vi "CTRE_Phoenix_MotorControl_ConfigBaseSettings.vi"(6 "timeoutMs":i32=50, 7 "Force Write":bool, 8 "error in (no error)":errorcluster, 10 "Base Configurables":T1={"openLoopRamp"=0.0, "closedLoopRamp"=0.0, "peakOutputForward"=1.0, "peakOutputReverse"=-1.0, "nominalOutputForward"=0.0, "nominalOutputReverse"=0.0, "neutralDeadband"=0.04, "voltageCompSaturation"=0.0, "voltageMeasurementFilter"=32, "velocityMeasurementPeriod"=100, "velocityMeasurementWindow"=64, "forwardSoftLimitThreshold"=0, "reverseSoftLimitThreshold"=0, "forwardSoftLimitEnable"=FALSE, "reverseSoftLimitEnable"=FALSE, "slot0"={"P"=0.0, "I"=0.0, "D"=0.0, "F"=0.0, "integralZone"=0.0, "allowableClosedLoopError"=0, "maxIntegralAccumulator"=0.0, "closedLoopPeakOutput"=1.0, "closedLoopPeriod"=1}, "slot1"={"P"=0.0, "I"=0.0, "D"=0.0, "F"=0.0, "integralZone"=0.0, "allowableClosedLoopError"=0, "maxIntegralAccumulator"=0.0, "closedLoopPeakOutput"=1.0, "closedLoopPeriod"=1}, "slot2"={"P"=0.0, "I"=0.0, "D"=0.0, "F"=0.0, "integralZone"=0.0, "allowableClosedLoopError"=0, "maxIntegralAccumulator"=0.0, "closedLoopPeakOutput"=1.0, "closedLoopPeriod"=1}, "slot3"={"P"=0.0, "I"=0.0, "D"=0.0, "F"=0.0, "integralZone"=0.0, "allowableClosedLoopError"=0, "maxIntegralAccumulator"=0.0, "closedLoopPeakOutput"=1.0, "closedLoopPeriod"=1}, "auxPIDPolarity"=FALSE, "remoteFilter0"={"remoteSensorDeviceID"=0, "remoteSensorSource"=enum."Off"}, "remoteFilter1"={"remoteSensorDeviceID"=0, "remoteSensorSource"=enum."Off"}, "motionCruiseVelocity"=0, "motionAcceleration"=0, "motionProfileTrajectoryPeriod"=0, "feedbackNotContinuous"=FALSE, "remoteSensorClosedLoopDisableNeutralOnLOS"=FALSE, "clearPositionOnLimitF"=FALSE, "clearPositionOnLimitR"=FALSE, "clearPositionOnQuadIdx"=FALSE, "limitSwitchDisableNeutralOnLOS"=FALSE, "softLimitDisableNeutralOnLOS"=FALSE, "pulseWidthPeriod_EdgesPerRot"=1, "pulseWidthPeriod_FilterWindowSz"=1, "customParam"={"customParam0"=0, "customParam1"=0}, "trajectoryInterpolationEnable"=TRUE} {"velocityMeasurementPeriod" items=["Period_1ms"=1, "Period_2ms"=2, "Period_5ms"=5, "Period_10ms"=10, "Period_20ms"=20, "Period_25ms"=25, "Period_50ms"=50, "Period_100ms"=100]}, 11 "PhoenixMotorControlDevRef in":T7) -> (0 "error out":errorcluster, 3 "PhoenixMotorControlDevRef out":T7)   [LabVIEW 2020]
doc: "Sets the base motor controller configurations for the selected motor controller"
uses:
  <vilib>/Rock Robotics/WPI/MotorControl/WPI_MotorControlDeviceRef.ctl
  <vilib>/Rock Robotics/WPI/MotorControl/WPI_MotorControlType.ctl
  <vilib>/Rock Robotics/SystemInterfaces/DIO/FPGA_DIOPWMChannel.ctl
  <vilib>/Rock Robotics/WPI/PWM/WPI_PWMDeadband.ctl
  <vilib>/Rock Robotics/SystemInterfaces/DIO/FPGA_DIOChannel.ctl
  <vilib>/Rock Robotics/WPI/ThirdParty/Phoenix-LabVIEW/Motor Controller/Controls/CTRE_Phoenix_MotorControl_BaseConfigurables.ctl
  <vilib>/Rock Robotics/WPI/ThirdParty/Phoenix-LabVIEW/Motor Controller/Controls/CTRE_Phoenix_MotorControl_VelocityMeasurementPeriod.ctl
  <vilib>/Rock Robotics/WPI/ThirdParty/Phoenix-LabVIEW/Motor Controller/Controls/CTRE_Phoenix_MotorControl_SlotStructure.ctl
  <vilib>/Rock Robotics/WPI/ThirdParty/Phoenix-LabVIEW/Motor Controller/Controls/CTRE_Phoenix_MotorControl_FilterStruct.ctl
  <vilib>/Rock Robotics/WPI/ThirdParty/Phoenix-LabVIEW/Motor Controller/Controls/CTRE_Phoenix_MotorControl_RemoteSourceType.ctl
  <vilib>/Rock Robotics/WPI/ThirdParty/Phoenix-LabVIEW/Controls/CTRE_Phoenix_CustomParamConfiguration.ctl
panel:
  # "False: Primary Output = PID[0] + PID[1]  ---  Auxiliary Output = PID[0] - PID[1]\nTrue:  Primary Output = PID[0] - PID[1] --- Auxiliary Output = PID[0] + PID[1]"
  # "Enable the motion profile executor to perform linear interpolation between profile points.  Defaults to True."
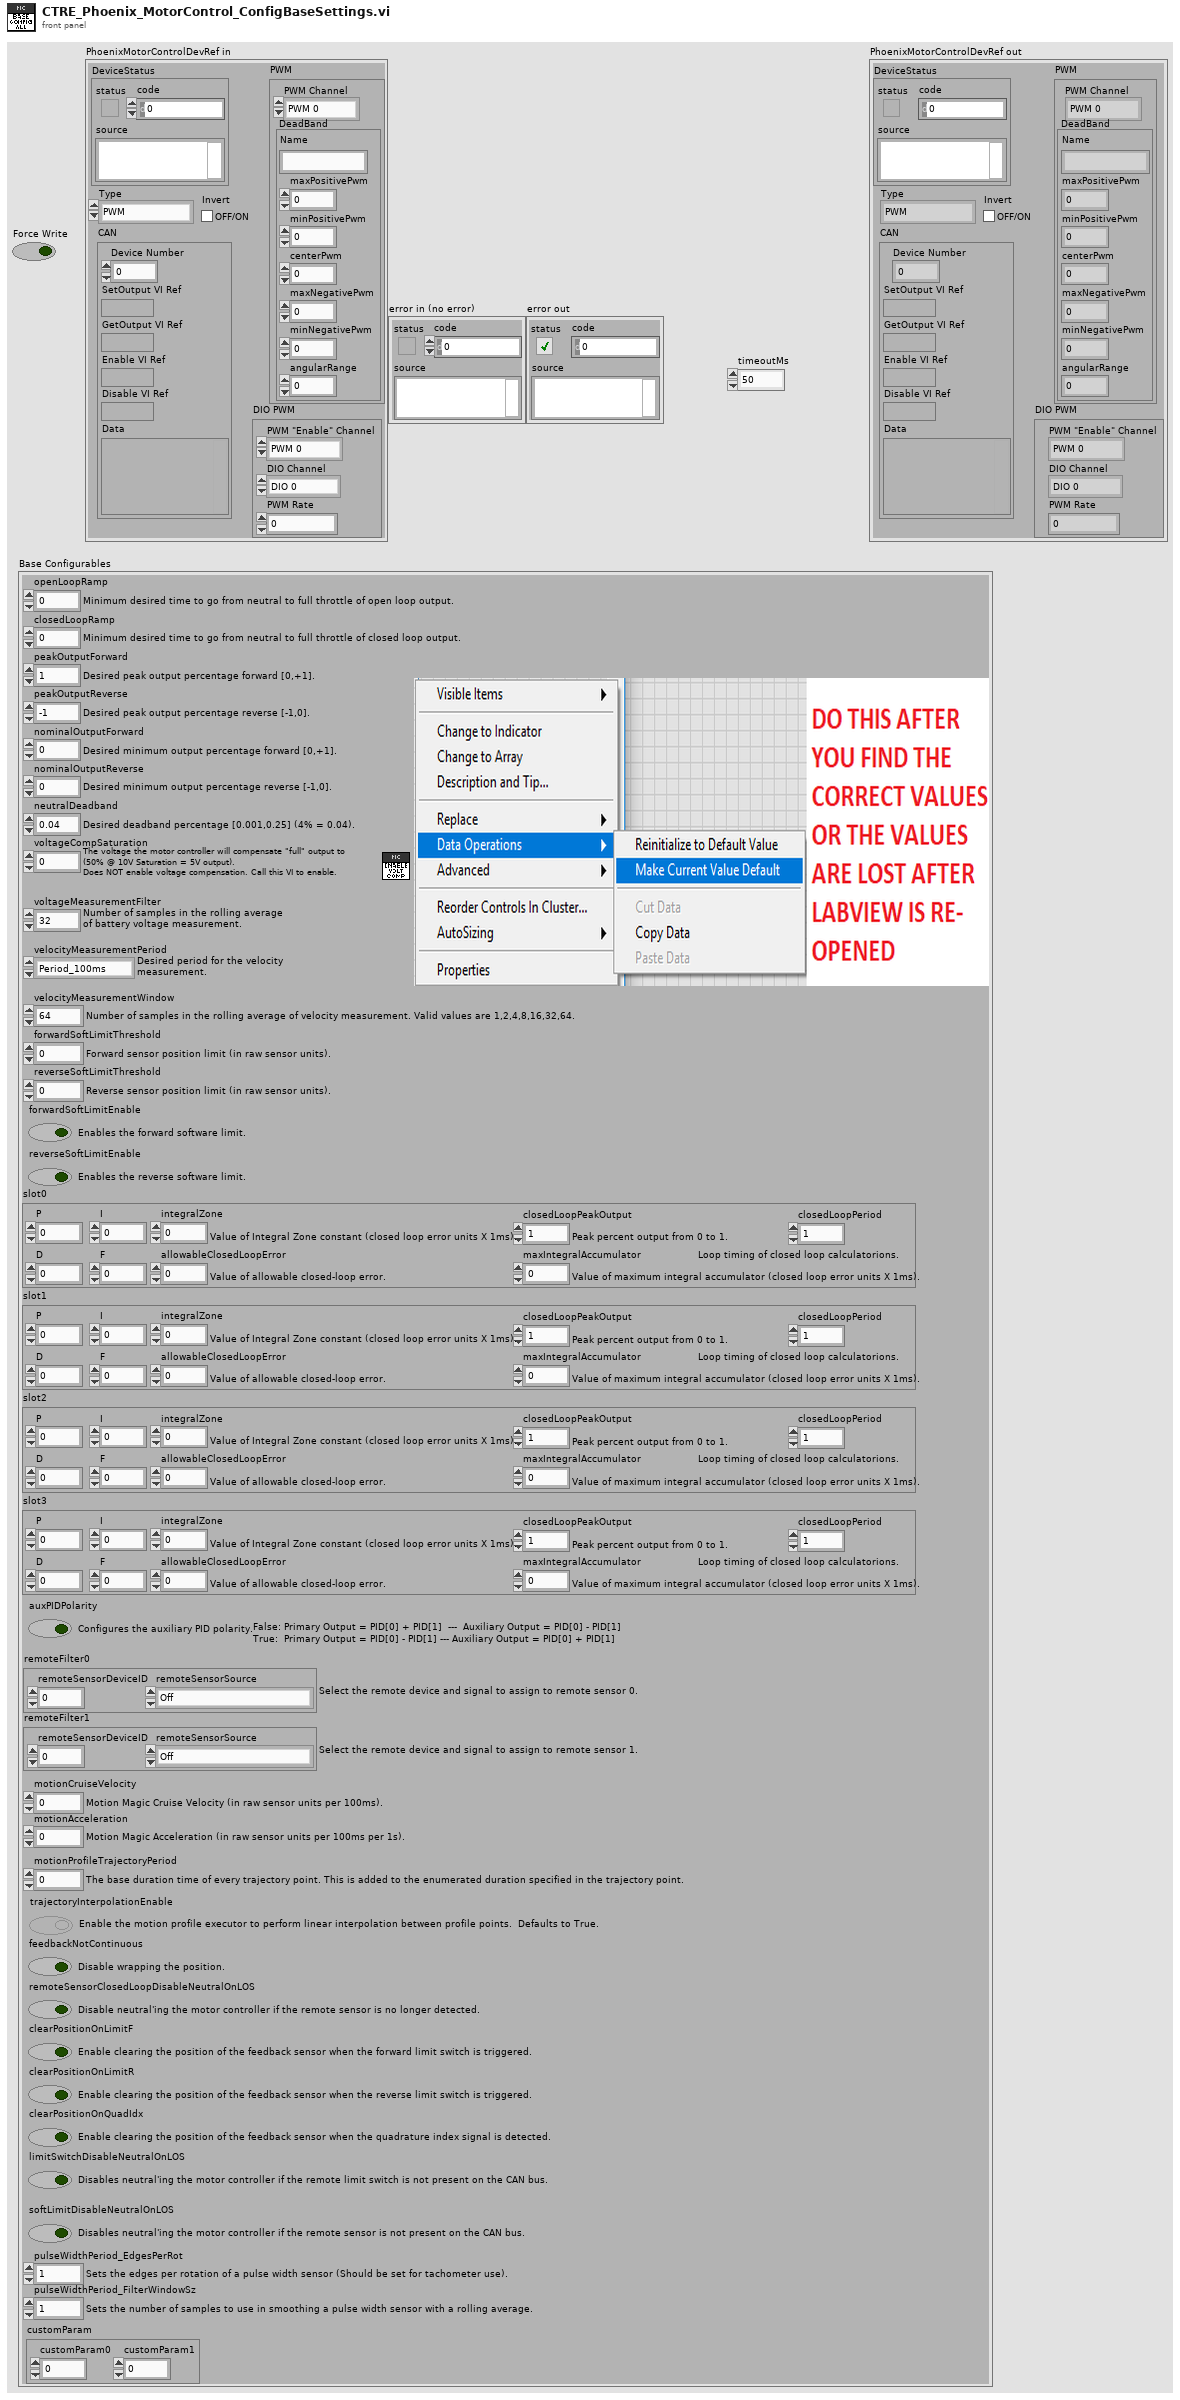
[diagram p1: front panel]
types:
  T1 = typedef "CTRE_Phoenix_MotorControl_BaseConfigurables.ctl" = cluster{"openLoopRamp":dbl, "closedLoopRamp":dbl, "peakOutputForward":dbl, "peakOutputReverse":dbl, "nominalOutputForward":dbl, "nominalOutputReverse":dbl, "neutralDeadband":dbl, "voltageCompSaturation":dbl, "voltageMeasurementFilter":i32, "velocityMeasurementPeriod":T2, "velocityMeasurementWindow":i32, "forwardSoftLimitThreshold":i32, "reverseSoftLimitThreshold":i32, "forwardSoftLimitEnable":bool, "reverseSoftLimitEnable":bool, "slot0":T3, "slot1":T3, "slot2":T3, "slot3":T3, "auxPIDPolarity":bool, "remoteFilter0":T4, "remoteFilter1":T4, "motionCruiseVelocity":i32, "motionAcceleration":i32, "motionProfileTrajectoryPeriod":i32, "feedbackNotContinuous":bool, "remoteSensorClosedLoopDisableNeutralOnLOS":bool, "clearPositionOnLimitF":bool, "clearPositionOnLimitR":bool, "clearPositionOnQuadIdx":bool, "limitSwitchDisableNeutralOnLOS":bool, "softLimitDisableNeutralOnLOS":bool, "pulseWidthPeriod_EdgesPerRot":i32, "pulseWidthPeriod_FilterWindowSz":i32, "customParam":T6, "trajectoryInterpolationEnable":bool}
  T2 = typedef "CTRE_Phoenix_MotorControl_VelocityMeasurementPeriod.ctl" = u16
  T3 = typedef "CTRE_Phoenix_MotorControl_SlotStructure.ctl" = cluster{"P":dbl, "I":dbl, "D":dbl, "F":dbl, "integralZone":dbl, "allowableClosedLoopError":i32, "maxIntegralAccumulator":dbl, "closedLoopPeakOutput":dbl, "closedLoopPeriod":i32}
  T4 = typedef "CTRE_Phoenix_MotorControl_FilterStruct.ctl" = cluster{"remoteSensorDeviceID":u8, "remoteSensorSource":T5}
  T5 = typedef "CTRE_Phoenix_MotorControl_RemoteSourceType.ctl" = enum16{"Off", "Talon SRX Selected Sensor", "Pigeon IMU Yaw", "Pigeon IMU Pitch", "Pigeon IMU Roll", "CANifier Quadrature", "CANifier PWM Input 0", "CANifier PWM Input 1", "CANifier PWM Input 2", "CANifier PWM Input 3", "Gadgeteer Pigeon Yaw", "Gadgeteer Pigeon Pitch", "Gadgeteer Pigeon Roll", "CANCoder"}
  T6 = typedef "CTRE_Phoenix_CustomParamConfiguration.ctl" = cluster{"customParam0":i32, "customParam1":i32}
  T7 = typedef "WPI_MotorControlDeviceRef.ctl" = cluster{"DeviceStatus":errorcluster, "Type":T8, "PWM":cluster{"PWM Channel":T9, "DeadBand":T10}, "CAN":cluster{"Device Number":u8, "SetOutput VI Ref":variant, "GetOutput VI Ref":variant, "Enable VI Ref":variant, "Disable VI Ref":variant, "Data":variant}, "Invert":bool, "DIO PWM":cluster{"PWM \"Enable\" Channel":T9, "DIOChannel":T11, "PWM Rate":dbl}}
  T8 = typedef "WPI_MotorControlType.ctl" = enum16{"PWM", "CAN", "DIO PWM"}
  T9 = typedef "FPGA_DIOPWMChannel.ctl" = enum8{"PWM 0", "PWM 1", "PWM 2", "PWM 3", "PWM 4", "PWM 5", "PWM 6", "PWM 7", "PWM 8", "PWM 9", "PWM MXP 0", "PWM MXP 1", "PWM MXP 2", "PWM MXP 3", "PWM MXP 4", "PWM MXP 5", "PWM MXP 6", "PWM MXP 7", "PWM MXP 8", "PWM MXP 9", "Invalid"}
  T10 = typedef "WPI_PWMDeadband.ctl" = cluster{"Name":string, "maxPositivePwm":i32, "minPositivePwm":i32, "centerPwm":i32, "maxNegativePwm":i32, "minNegativePwm":i32, "angularRange":u16}
  T11 = typedef "FPGA_DIOChannel.ctl" = enum8{"DIO 0", "DIO 1", "DIO 2", "DIO 3", "DIO 4", "DIO 5", "DIO 6", "DIO 7", "DIO 8", "DIO 9", "DIO MXP 0", "DIO MXP 1", "DIO MXP 2", "DIO MXP 3", "DIO MXP 4", "DIO MXP 5", "DIO MXP 6", "DIO MXP 7", "DIO MXP 8", "DIO MXP 9", "DIO MXP 10", "DIO MXP 11", "DIO MXP 12", "DIO MXP 13", "DIO MXP 14", "DIO MXP 15", "SPI Port CS1", "SPI Port CS2", "SPI Port CS3", "SPI Port MISO", "SPI Port MOSI", "Invalid"}
  T12 = cluster{"openLoopRamp":bool, "closedLoopRamp":bool, "peakOutputForward":bool, "peakOutputReverse":bool, "nominalOutputForward":bool, "nominalOutputReverse":bool, "neutralDeadband":bool, "voltageCompSaturation":bool, "voltageMeasurementFilter":bool, "velocityMeasurementPeriod":bool, "velocityMeasurementWindow":bool, "forwardSoftLimitThreshold":bool, "reverseSoftLimitThreshold":bool, "forwardSoftLimitEnable":bool, "reverseSoftLimitEnable":bool, "slot0":cluster{"P":bool, "I":bool, "D":bool, "F":bool, "integralZone":bool, "allowableClosedLoopError":bool, "maxIntegralAccumulator":bool, "closedLoopPeakOutput":bool, "closedLoopPeriod":bool}, "slot1":cluster{"P":bool, "I":bool, "D":bool, "F":bool, "integralZone":bool, "allowableClosedLoopError":bool, "maxIntegralAccumulator":bool, "closedLoopPeakOutput":bool, "closedLoopPeriod":bool}, "slot2":cluster{"P":bool, "I":bool, "D":bool, "F":bool, "integralZone":bool, "allowableClosedLoopError":bool, "maxIntegralAccumulator":bool, "closedLoopPeakOutput":bool, "closedLoopPeriod":bool}, "slot3":cluster{"P":bool, "I":bool, "D":bool, "F":bool, "integralZone":bool, "allowableClosedLoopError":bool, "maxIntegralAccumulator":bool, "closedLoopPeakOutput":bool, "closedLoopPeriod":bool}, "auxPIDPolarity":bool, "remoteFilter0":cluster{"remoteSensorDeviceID":bool, "remoteSensorSource":bool}, "remoteFilter1":cluster{"remoteSensorDeviceID":bool, "remoteSensorSource":bool}, "motionCruiseVelocity":bool, "motionAcceleration":bool, "motionProfileTrajectoryPeriod":bool, "feedbackNotContinuous":bool, "remoteSensorClosedLoopDisableNeutralOnLOS":bool, "clearPositionOnLimitF":bool, "clearPositionOnLimitR":bool, "clearPositionOnQuadIdx":bool, "limitSwitchDisableNeutralOnLOS":bool, "softLimitDisableNeutralOnLOS":bool, "pulseWidthPeriod_EdgesPerRot":bool, "pulseWidthPeriod_FilterWindowSz":bool, "customParam":cluster{"customParam0":bool, "customParam1":bool}, "trajectoryInterpolationEnable":bool}
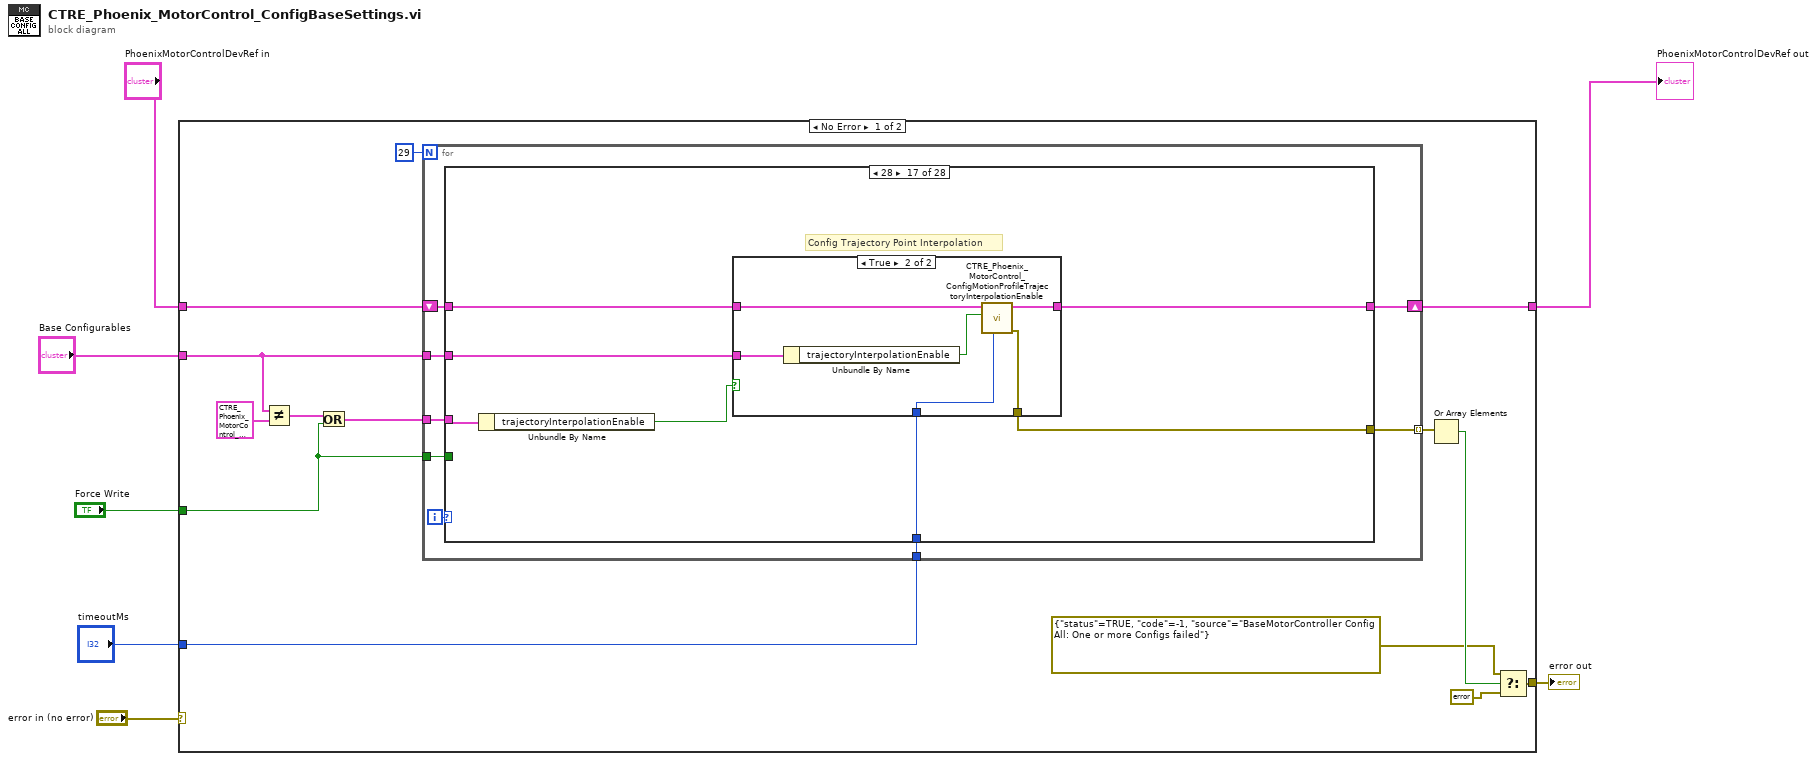
[diagram p0: block diagram]
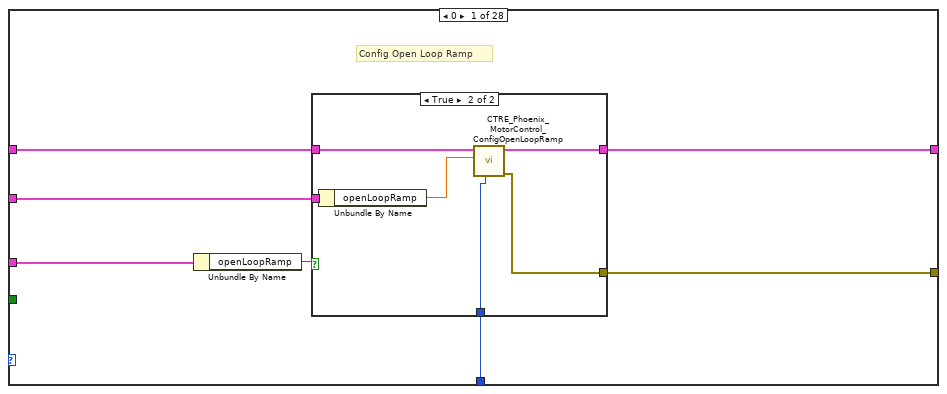
[diagram p2: hidden frame]
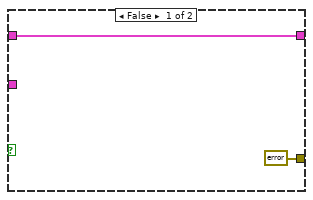
[diagram p3: hidden frame]
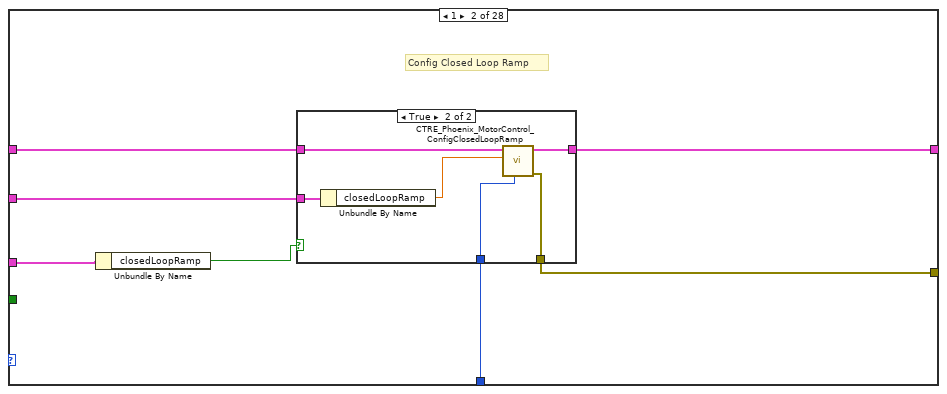
[diagram p4: hidden frame]
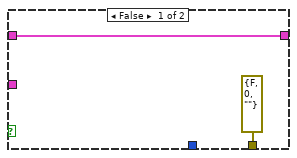
[diagram p5: hidden frame]
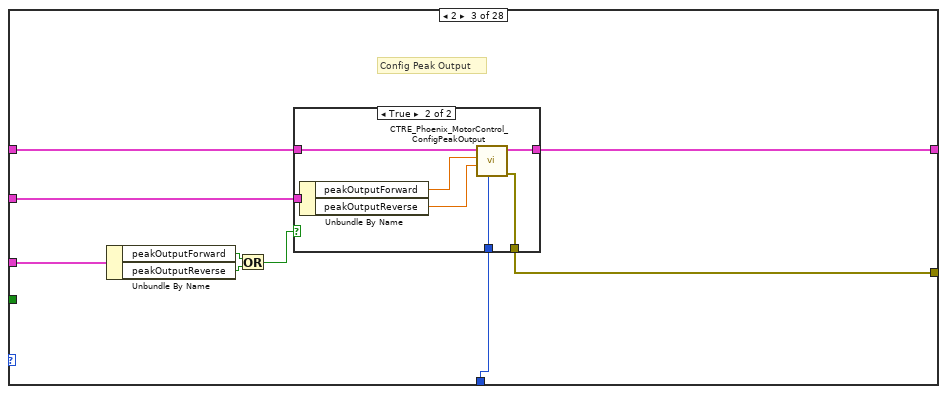
[diagram p6: hidden frame]
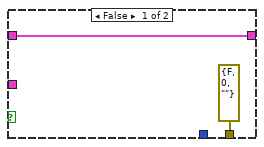
[diagram p7: hidden frame]
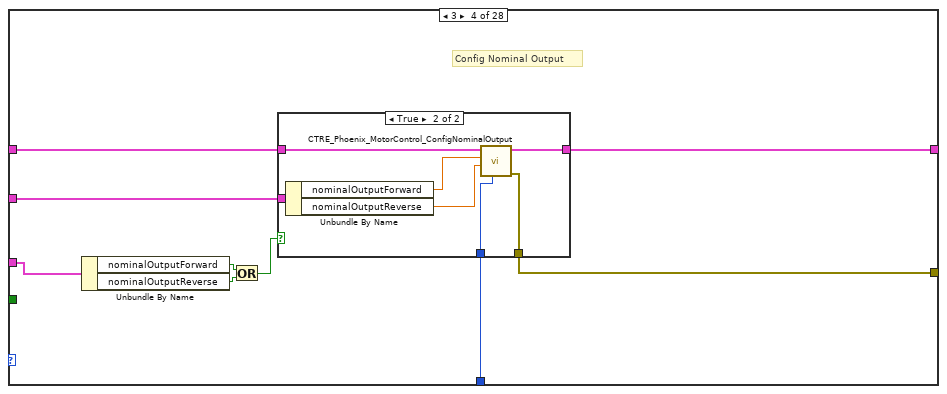
[diagram p8: hidden frame]
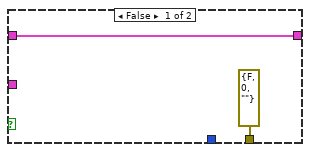
[diagram p9: hidden frame]
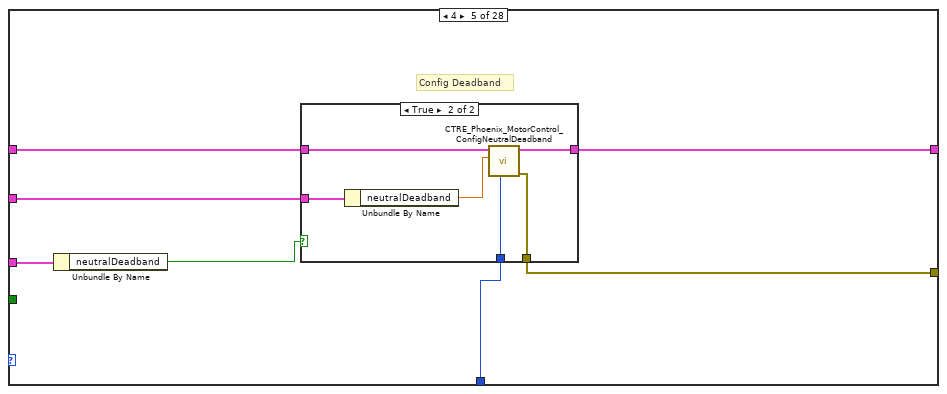
[diagram p10: hidden frame]
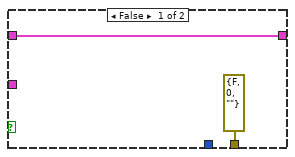
[diagram p11: hidden frame]
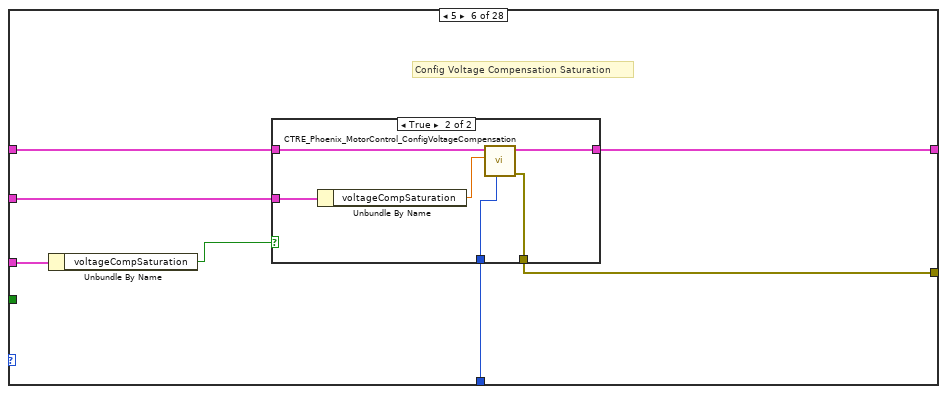
[diagram p12: hidden frame]
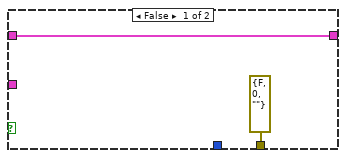
[diagram p13: hidden frame]
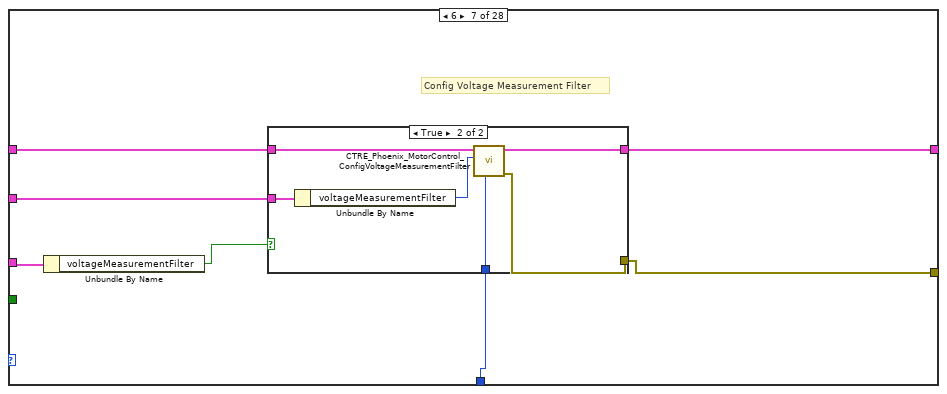
[diagram p14: hidden frame]
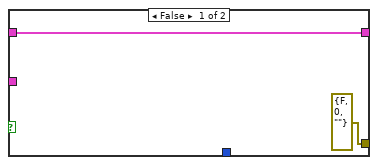
[diagram p15: hidden frame]
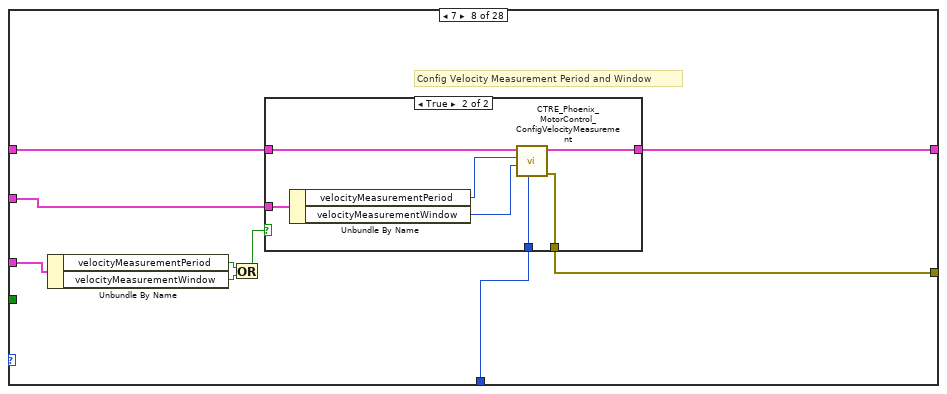
[diagram p16: hidden frame]
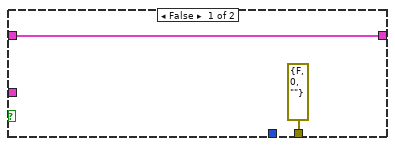
[diagram p17: hidden frame]
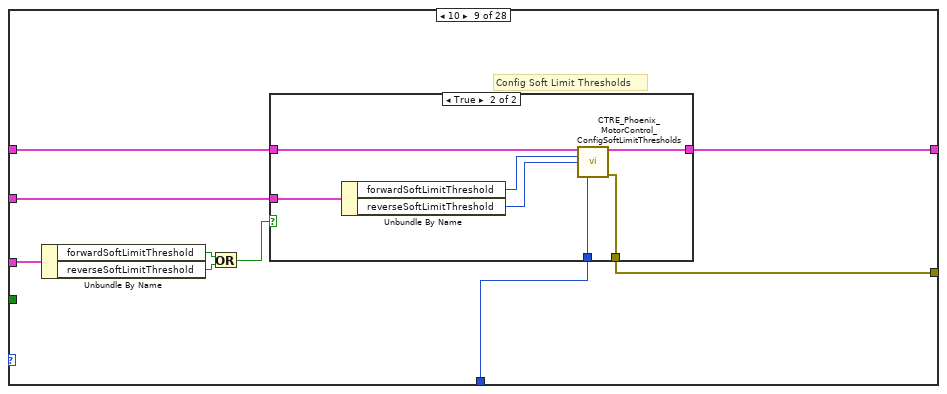
[diagram p18: hidden frame]
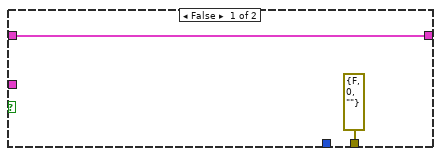
[diagram p19: hidden frame]
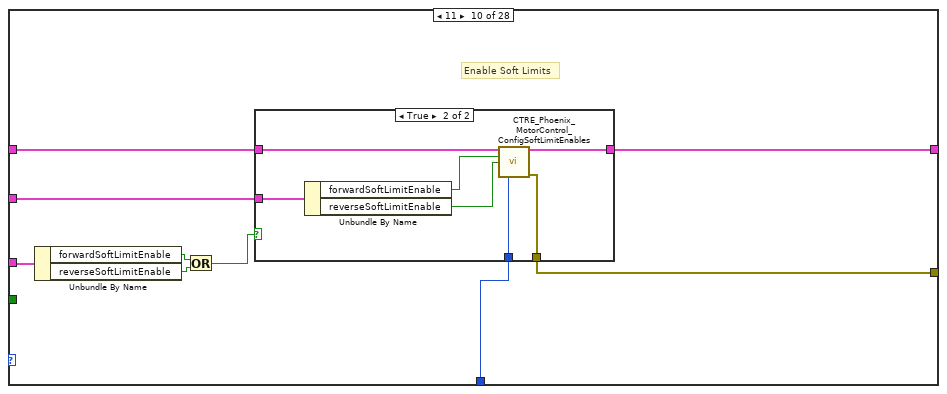
[diagram p20: hidden frame]
diagram:
  n1 = case shown="No Error" "error in (no error)" {
    selector: "error in (no error)" -> [_ w467]
    tunnel: "timeoutMs" -> [w19 _]
    tunnel: [w18 w468] -> w6
    tunnel: "PhoenixMotorControlDevRef in" -> [w17 w468]
    tunnel: "Base Configurables" -> [w16 _]
    tunnel: "Force Write" -> [w12 _]
    tunnel: [w8 w467] -> w1
    frame No Error {
      n2 = Not Equal?(x=w16, y=T1 {"openLoopRamp"=0.0, "closedLoopRamp"=0.0, "peakOutputForward"=1.0, "peakOutputReverse"=-1.0, "nominalOutputForward"=0.0, "nominalOutputReverse"=0.0, "neutralDeadband"=0.04, "voltageCompSaturation"=0.0, "voltageMeasurementFilter"=32, "velocityMeasurementPeriod"=100, "velocityMeasurementWindow"=64, "forwardSoftLimitThreshold"=0, "reverseSoftLimitThreshold"=0, "forwardSoftLimitEnable"=FALSE, "reverseSoftLimitEnable"=FALSE, "slot0"={"P"=0.0, "I"=0.0, "D"=0.0, "F"=0.0, "integralZone"=0.0, "allowableClosedLoopError"=0, "maxIntegralAccumulator"=0.0, "closedLoopPeakOutput"=1.0, "closedLoopPeriod"=1}, "slot1"={"P"=0.0, "I"=0.0, "D"=0.0, "F"=0.0, "integralZone"=0.0, "allowableClosedLoopError"=0, "maxIntegralAccumulator"=0.0, "closedLoopPeakOutput"=1.0, "closedLoopPeriod"=1}, "slot2"={"P"=0.0, "I"=0.0, "D"=0.0, "F"=0.0, "integralZone"=0.0, "allowableClosedLoopError"=0, "maxIntegralAccumulator"=0.0, "closedLoopPeakOutput"=1.0, "closedLoopPeriod"=1}, "slot3"={"P"=0.0, "I"=0.0, "D"=0.0, "F"=0.0, "integralZone"=0.0, "allowableClosedLoopError"=0, "maxIntegralAccumulator"=0.0, "closedLoopPeakOutput"=1.0, "closedLoopPeriod"=1}, "auxPIDPolarity"=FALSE, "remoteFilter0"={"remoteSensorDeviceID"=0, "remoteSensorSource"=enum."Off"}, "remoteFilter1"={"remoteSensorDeviceID"=0, "remoteSensorSource"=enum."Off"}, "motionCruiseVelocity"=0, "motionAcceleration"=0, "motionProfileTrajectoryPeriod"=0, "feedbackNotContinuous"=FALSE, "remoteSensorClosedLoopDisableNeutralOnLOS"=FALSE, "clearPositionOnLimitF"=FALSE, "clearPositionOnLimitR"=FALSE, "clearPositionOnQuadIdx"=FALSE, "limitSwitchDisableNeutralOnLOS"=FALSE, "softLimitDisableNeutralOnLOS"=FALSE, "pulseWidthPeriod_EdgesPerRot"=1, "pulseWidthPeriod_FilterWindowSz"=1, "customParam"={"customParam0"=0, "customParam1"=0}, "trajectoryInterpolationEnable"=TRUE}) -> (x != y?=w14:T12)
      n3 = Or(x=w14, y=w12) -> (x .or. y?=w13:T12)
      n4 = for {
        N: 29 -> [_]
        tunnel: w19 -> [w27]
        tunnel: w16 -> [w26]
        shift-right: [w28] -> w18
        shift-left: w17 -> [w29]
        tunnel: [w24] -> w20 mode=indexing
        tunnel: w13 -> [w23]
        tunnel: w12 -> [w22]
        i -> [w25]
        n5 = case shown="28" w25 {
          tunnel: w29 -> [w35 w49 w67 w85 w101 w116 w131 w148 w166 w185 w202 w226 w243 w262 w281 w297 w312 w327 w342 w357 w372 w387 w402 w417 w432 w447 w463 w466]
          tunnel: [w34 w50 w66 w84 w100 w115 w130 w147 w165 w184 w201 w225 w242 w263 w280 w296 w311 w326 w341 w356 w371 w386 w400 w416 w431 w446 w462 w466] -> w28
          tunnel: w27 -> [w33 w48 w64 w82 w99 w114 w129 w146 w164 w182 w199 w224 w241 w260 w279 w295 w310 w325 w340 w355 w370 w385 w401 w415 w429 w445 w461 _]
          tunnel: w26 -> [w36 w51 w68 w86 w102 w117 w132 w149 w167 w183 w204 w227 w244 w261 w282 w298 w313 w328 w343 w358 w373 w388 w403 w418 w433 w448 w464 _]
          tunnel: [w32 w47 w65 w83 w98 w113 w128 w145 w163 w181 w197 w223 w240 w259 w278 w294 w309 w324 w339 w354 w369 w384 w399 w414 w430 w444 w457 errorcluster {"status"=FALSE, "code"=0, "source"=""} ("error out")] -> w24
          tunnel: w23 -> [w31 w46 w63 w81 w97 w112 w127 w144 w162 w180 _ w222 w239 w258 w277 w293 w308 w323 w338 w353 w368 w383 w398 w413 w428 w442 _ _]
          tunnel: w22 -> [_ _ _ _ _ _ _ _ _ _ w195 _ _ _ _ _ _ _ _ _ _ _ _ _ _ _ _ _]
          frame 0 {
            # "Config Open Loop Ramp"
            n6 = Unbundle By Name(w31) -> ("openLoopRamp"=w30:bool)
            n7 = case shown="True" w30 {
              tunnel: w36 -> [_ w44]
              tunnel: w35 -> [w38 w43]
              tunnel: [w38 w42] -> w34
              tunnel: w33 -> [_ w40]
              tunnel: [errorcluster {"status"=FALSE, "code"=0, "source"=""} ("error out") w39] -> w32
              frame False {
              }
              frame True {
                n8 = Unbundle By Name(w44) -> ("openLoopRamp"=w41:dbl)
                n9 = call <vilib>:"CTRE_Phoenix_MotorControl_ConfigOpenLoopRamp.vi"("timeoutMs"=w40, "secondsFromNeutralToFull"=w41, "PhoenixMotorControlDevRef"=w43) -> ("error out"=w39:errorcluster, "PhoenixMotorControlDevRef"=w42:T7)  [unwired: 7 in]
              }
            }
          }
          frame 1 {
            # "Config Closed Loop Ramp"
            n10 = Unbundle By Name(w46) -> ("closedLoopRamp"=w45:bool)
            n11 = case shown="True" w45 {
              tunnel: w51 -> [_ w59]
              tunnel: [w53 w58] -> w50
              tunnel: w49 -> [w53 w57]
              tunnel: w48 -> [_ w55]
              tunnel: [errorcluster {"status"=FALSE, "code"=0, "source"=""} ("error out") w54] -> w47
              frame False {
              }
              frame True {
                n12 = Unbundle By Name(w59) -> ("closedLoopRamp"=w56:dbl)
                n13 = call <vilib>:"CTRE_Phoenix_MotorControl_ConfigClosedLoopRamp.vi"("timeoutMs"=w55, "secondsFromNeutralToFull"=w56, "PhoenixMotorControlDevRef"=w57) -> ("error out"=w54:errorcluster, "PhoenixMotorControlDevRef"=w58:T7)  [unwired: 7 in]
              }
            }
          }
          frame 2 {
            # "Config Peak Output"
            n14 = Unbundle By Name(w63) -> ("peakOutputForward"=w61:bool, "peakOutputReverse"=w62:bool)
            n15 = Or(x=w61, y=w62) -> (x .or. y?=w60:bool)
            n16 = case shown="True" w60 {
              tunnel: w68 -> [_ w77]
              tunnel: w67 -> [w70 w76]
              tunnel: [w70 w75] -> w66
              tunnel: [errorcluster {"status"=FALSE, "code"=0, "source"=""} ("error out") w72] -> w65
              tunnel: w64 -> [_ w71]
              frame False {
              }
              frame True {
                n17 = Unbundle By Name(w77) -> ("peakOutputForward"=w74:dbl, "peakOutputReverse"=w73:dbl)
                n18 = call <vilib>:"CTRE_Phoenix_MotorControl_ConfigPeakOutput.vi"("timeoutMs"=w71, "Reverse Peak Percent Output"=w73, "Forward Peak Percent Output"=w74, "PhoenixMotorControlDevRef"=w76) -> ("error out"=w72:errorcluster, "PhoenixMotorControlDevRef"=w75:T7)  [unwired: 6 in]
              }
            }
          }
          frame 3 {
            # "Config Nominal Output"
            n19 = Unbundle By Name(w81) -> ("nominalOutputForward"=w79:bool, "nominalOutputReverse"=w80:bool)
            n20 = Or(x=w79, y=w80) -> (x .or. y?=w78:bool)
            n21 = case shown="True" w78 {
              tunnel: w86 -> [_ w95]
              tunnel: w85 -> [w88 w94]
              tunnel: [w88 w93] -> w84
              tunnel: [errorcluster {"status"=FALSE, "code"=0, "source"=""} ("error out") w90] -> w83
              tunnel: w82 -> [_ w89]
              frame False {
              }
              frame True {
                n22 = Unbundle By Name(w95) -> ("nominalOutputForward"=w92:dbl, "nominalOutputReverse"=w91:dbl)
                n23 = call <vilib>:"CTRE_Phoenix_MotorControl_ConfigNominalOutput.vi"("timeoutMs"=w89, "Reverse Nominal Percent Output"=w91, "Forward Nominal Percent Output"=w92, "PhoenixMotorControlDevRef"=w94) -> ("error out"=w90:errorcluster, "PhoenixMotorControlDevRef"=w93:T7)  [unwired: 6 in]
              }
            }
          }
          frame 4 {
            # "Config Deadband"
            n24 = Unbundle By Name(w97) -> ("neutralDeadband"=w96:bool)
            n25 = case shown="True" w96 {
              tunnel: w102 -> [_ w110]
              tunnel: w101 -> [w104 w109]
              tunnel: [w104 w108] -> w100
              tunnel: w99 -> [_ w106]
              tunnel: [errorcluster {"status"=FALSE, "code"=0, "source"=""} ("error out") w105] -> w98
              frame False {
              }
              frame True {
                n26 = Unbundle By Name(w110) -> ("neutralDeadband"=w107:dbl)
                n27 = call <vilib>:"CTRE_Phoenix_MotorControl_ConfigNeutralDeadband.vi"("timeoutMs"=w106, "Percent Deadband"=w107, "PhoenixMotorControlDevRef"=w109) -> ("error out"=w105:errorcluster, "PhoenixMotorControlDevRef"=w108:T7)  [unwired: 7 in]
              }
            }
          }
          frame 5 {
            # "Config Voltage Compensation Saturation"
            n28 = Unbundle By Name(w112) -> ("voltageCompSaturation"=w111:bool)
            n29 = case shown="True" w111 {
              tunnel: w117 -> [_ w125]
              tunnel: w116 -> [w119 w124]
              tunnel: [w119 w123] -> w115
              tunnel: w114 -> [_ w121]
              tunnel: [errorcluster {"status"=FALSE, "code"=0, "source"=""} ("error out") w120] -> w113
              frame False {
              }
              frame True {
                n30 = Unbundle By Name(w125) -> ("voltageCompSaturation"=w122:dbl)
                n31 = call <vilib>:"CTRE_Phoenix_MotorControl_ConfigVoltageCompensation.vi"("timeoutMs"=w121, "Saturation Voltage"=w122, "PhoenixMotorControlDevRef"=w124) -> ("error out"=w120:errorcluster, "PhoenixMotorControlDevRef"=w123:T7)  [unwired: 7 in]
              }
            }
          }
          frame 6 {
            # "Config Voltage Measurement Filter"
            n32 = Unbundle By Name(w127) -> ("voltageMeasurementFilter"=w126:bool)
            n33 = case shown="True" w126 {
              tunnel: w132 -> [_ w140]
              tunnel: w131 -> [w134 w139]
              tunnel: [w134 w138] -> w130
              tunnel: w129 -> [_ w136]
              tunnel: [errorcluster {"status"=FALSE, "code"=0, "source"=""} ("error out") w135] -> w128
              frame False {
              }
              frame True {
                n34 = Unbundle By Name(w140) -> ("voltageMeasurementFilter"=w137:i32)
                n35 = call <vilib>:"CTRE_Phoenix_MotorControl_ConfigVoltageMeasurementFilter.vi"("timeoutMs"=w136, "filterWindowSamples"=w137, "PhoenixMotorControlDevRef"=w139) -> ("error out"=w135:errorcluster, "PhoenixMotorControlDevRef"=w138:T7)  [unwired: 7 in]
              }
            }
          }
          frame 7 {
            # "Config Velocity Measurement Period and Window"
            n36 = Unbundle By Name(w144) -> ("velocityMeasurementPeriod"=w142:bool, "velocityMeasurementWindow"=w143:bool)
            n37 = Or(x=w142, y=w143) -> (x .or. y?=w141:bool)
            n38 = case shown="True" w141 {
              tunnel: w149 -> [_ w158]
              tunnel: w148 -> [w151 w157]
              tunnel: [w151 w156] -> w147
              tunnel: w146 -> [_ w153]
              tunnel: [errorcluster {"status"=FALSE, "code"=0, "source"=""} ("error out") w152] -> w145
              frame False {
              }
              frame True {
                n39 = Unbundle By Name(w158) -> ("velocityMeasurementPeriod"=w155:T2, "velocityMeasurementWindow"=w154:i32)
                n40 = call <vilib>:"CTRE_Phoenix_MotorControl_ConfigVelocityMeasurement.vi"("timeoutMs"=w153, "Window Size"=w154, "Velocity Measurement Period"=w155, "PhoenixMotorControlDevRef"=w157) -> ("error out"=w152:errorcluster, "PhoenixMotorControlDevRef"=w156:T7)  [unwired: 6 in]
              }
            }
          }
          frame 10 {
            # "Config Soft Limit Thresholds"
            n41 = Unbundle By Name(w162) -> ("forwardSoftLimitThreshold"=w160:bool, "reverseSoftLimitThreshold"=w161:bool)
            n42 = Or(x=w160, y=w161) -> (x .or. y?=w159:bool)
            n43 = case shown="True" w159 {
              tunnel: w167 -> [_ w176]
              tunnel: w166 -> [w169 w175]
              tunnel: [w169 w174] -> w165
              tunnel: w164 -> [_ w171]
              tunnel: [errorcluster {"status"=FALSE, "code"=0, "source"=""} ("error out") w170] -> w163
              frame False {
              }
              frame True {
                n44 = Unbundle By Name(w176) -> ("forwardSoftLimitThreshold"=w173:i32, "reverseSoftLimitThreshold"=w172:i32)
                n45 = call <vilib>:"CTRE_Phoenix_MotorControl_ConfigSoftLimitThresholds.vi"("PhoenixMotorControlDevRef"=w175, "Forward Soft Limit"=w173, "Reverse Soft Limit"=w172, "timeoutMs"=w171) -> ("PhoenixMotorControlDevRef"=w174:T7, "error out"=w170:errorcluster)  [unwired: 10 in]
              }
            }
          }
          frame 11 {
            # "Enable Soft Limits"
            n46 = Unbundle By Name(w180) -> ("forwardSoftLimitEnable"=w178:bool, "reverseSoftLimitEnable"=w179:bool)
            n47 = Or(x=w178, y=w179) -> (x .or. y?=w177:bool)
            n48 = case shown="True" w177 {
              tunnel: w185 -> [w187 w194]
              tunnel: [w187 w193] -> w184
              tunnel: w183 -> [_ w192]
              tunnel: w182 -> [_ w189]
              tunnel: [errorcluster {"status"=FALSE, "code"=0, "source"=""} ("error out") w188] -> w181
              frame False {
              }
              frame True {
                n49 = Unbundle By Name(w192) -> ("forwardSoftLimitEnable"=w191:bool, "reverseSoftLimitEnable"=w190:bool)
                n50 = call <vilib>:"CTRE_Phoenix_MotorControl_ConfigSoftLimitEnables.vi"("PhoenixMotorControlDevRef"=w194, "Forward Soft Limit Enable"=w191, "Reverse Soft Limit Enable"=w190, "timeoutMs"=w189) -> ("PhoenixMotorControlDevRef"=w193:T7, "error out"=w188:errorcluster)  [unwired: 10 in]
              }
            }
          }
          frame 12 {
            # "Configure the 4 slots"
            n51 = for {
              N: 4 -> [_]
              tunnel: w204 -> [w212]
              shift-right: [w211] -> w201
              shift-left: w202 -> [w209]
              tunnel: [w206] -> w200 mode=indexing
              tunnel: w199 -> [w210]
              tunnel: w195 -> [w205]
              i -> [w207]
              n52 = case shown="3" w207 {
                tunnel: w212 -> [w214 w216 w218 w220]
                tunnel: [w213 w215 w217 w219] -> w208
                frame 3 {
                  n53 = Unbundle By Name(w214) -> ("slot3"=w213:T3)
                }
                frame 0, Default {
                  n54 = Unbundle By Name(w216) -> ("slot0"=w215:T3)
                }
                frame 1 {
                  n55 = Unbundle By Name(w218) -> ("slot1"=w217:T3)
                }
                frame 2 {
                  n56 = Unbundle By Name(w220) -> ("slot2"=w219:T3)
                }
              }
              n57 = call <vilib>:"CTRE_Phoenix_MotorControl_ConfigSlot.vi"("timeoutMs"=w210, "Force Write"=w205, "Slot Number"=w207, "Slot Struct"=w208, "PhoenixMotorControlDevRef"=w209) -> ("error out"=w206:errorcluster, "PhoenixMotorControlDevRef"=w211:T7)  [unwired: 5 in]
            }
            n58 = Or Array Elements(Boolean array=w200) -> (logical OR=w198:bool)
            n59 = Bundle By Name(cluster=errorcluster {"status"=TRUE, "code"=0, "source"=""} ("error out 2"), "status"=w198) -> (w197:errorcluster)
          }
          frame 13 {
            # "Config Auxiliary PID Polarity"
            n60 = Unbundle By Name(w222) -> ("auxPIDPolarity"=w221:bool)
            n61 = case shown="True" w221 {
              tunnel: w227 -> [_ w235]
              tunnel: w226 -> [w229 w234]
              tunnel: [w229 w233] -> w225
              tunnel: w224 -> [_ w231]
              tunnel: [errorcluster {"status"=FALSE, "code"=0, "source"=""} ("error out") w230] -> w223
              frame False {
              }
              frame True {
                n62 = Unbundle By Name(w235) -> ("auxPIDPolarity"=w232:bool)
                n63 = call <vilib>:"CTRE_Phoenix_MotorControl_ConfigAuxPolarity.vi"("timeoutMs"=w231, "Invert"=w232, "PhoenixMotorControlDevRef"=w234) -> ("error out"=w230:errorcluster, "PhoenixMotorControlDevRef"=w233:T7)  [unwired: 7 in]
              }
            }
          }
          frame 14 {
            n64 = Unbundle By Name(w239) -> ("remoteFilter0.remoteSensorSource"=w237:bool, "remoteFilter0.remoteSensorDeviceID"=w238:bool)
            n65 = Or(x=w237, y=w238) -> (x .or. y?=w236:bool)
            n66 = case shown="True" w236 {
              tunnel: w244 -> [_ w254]
              tunnel: w243 -> [w246 w253]
              tunnel: [w246 w252] -> w242
              tunnel: w241 -> [_ w248]
              tunnel: [errorcluster {"status"=FALSE, "code"=0, "source"=""} ("error out") w247] -> w240
              frame False {
              }
              frame True {
                # "Config Remote Sensor 0"
                n67 = Unbundle By Name(w254) -> ("remoteFilter0.remoteSensorSource"=w251:T5, "remoteFilter0.remoteSensorDeviceID"=w250:u8)
                n68 = call <vilib>:"CTRE_Phoenix_MotorControl_ConfigRemoteSource.vi"("PhoenixMotorControlDevRef"=w253, "Remote Device Type"=w251, "Remote Device ID"=w250, "Source Index (0/1)"=u32 0, "timeoutMs"=w248) -> ("PhoenixMotorControlDevRef"=w252:T7, "error out"=w247:errorcluster)  [unwired: 9 in]
              }
            }
          }
          frame 15 {
            # "Config Remote Sensor 1"
            n69 = Unbundle By Name(w258) -> ("remoteFilter1.remoteSensorSource"=w256:bool, "remoteFilter1.remoteSensorDeviceID"=w257:bool)
            n70 = Or(x=w256, y=w257) -> (x .or. y?=w255:bool)
            n71 = case shown="True" w255 {
              tunnel: [w264 w270] -> w263
              tunnel: w262 -> [w264 w269]
              tunnel: w261 -> [_ w268]
              tunnel: w260 -> [_ w267]
              tunnel: [errorcluster {"status"=FALSE, "code"=0, "source"=""} ("error out") w266] -> w259
              frame False {
              }
              frame True {
                n72 = Unbundle By Name(w268) -> ("remoteFilter1.remoteSensorSource"=w273:T5, "remoteFilter1.remoteSensorDeviceID"=w272:u8)
                n73 = call <vilib>:"CTRE_Phoenix_MotorControl_ConfigRemoteSource.vi"("PhoenixMotorControlDevRef"=w269, "Remote Device Type"=w273, "Remote Device ID"=w272, "Source Index (0/1)"=u32 1, "timeoutMs"=w267) -> ("PhoenixMotorControlDevRef"=w270:T7, "error out"=w266:errorcluster)  [unwired: 9 in]
              }
            }
          }
          frame 16 {
            # "Config Motion Magic"
            n74 = Unbundle By Name(w277) -> ("motionCruiseVelocity"=w275:bool, "motionAcceleration"=w276:bool)
            n75 = Or(x=w275, y=w276) -> (x .or. y?=w274:bool)
            n76 = case shown="True" w274 {
              tunnel: w282 -> [_ w291]
              tunnel: w281 -> [w283 w290]
              tunnel: [w283 w289] -> w280
              tunnel: w279 -> [_ w286]
              tunnel: [errorcluster {"status"=FALSE, "code"=0, "source"=""} ("error out") w285] -> w278
              frame False {
              }
              frame True {
                n77 = Unbundle By Name(w291) -> ("motionCruiseVelocity"=w288:i32, "motionAcceleration"=w287:i32)
                n78 = call <vilib>:"CTRE_Phoenix_MotorControl_ConfigMotionMagic.vi"("timeoutMs"=w286, "Acceleration"=w287, "Cruise Velocity"=w288, "PhoenixMotorControlDevRef"=w290) -> ("error out"=w285:errorcluster, "PhoenixMotorControlDevRef"=w289:T7)  [unwired: 6 in]
              }
            }
          }
          frame 17 {
            # "Config Global Trajectory Point Duration"
            n79 = Unbundle By Name(w293) -> ("motionProfileTrajectoryPeriod"=w292:bool)
            n80 = case shown="True" w292 {
              tunnel: w298 -> [_ w306]
              tunnel: w297 -> [w300 w305]
              tunnel: [w300 w304] -> w296
              tunnel: w295 -> [_ w302]
              tunnel: [errorcluster {"status"=FALSE, "code"=0, "source"=""} ("error out") w301] -> w294
              frame False {
              }
              frame True {
                n81 = Unbundle By Name(w306) -> ("motionProfileTrajectoryPeriod"=w303:i32)
                n82 = call <vilib>:"CTRE_Phoenix_MotorControl_ConfigTrajectoryPointDuration.vi"("timeoutMs"=w302, "durationMs"=w303, "PhoenixMotorControlDevRef"=w305) -> ("error out"=w301:errorcluster, "PhoenixMotorControlDevRef"=w304:T7)  [unwired: 7 in]
              }
            }
          }
          frame 28 {
            # "Config Trajectory Point Interpolation"
            n83 = Unbundle By Name(w308) -> ("trajectoryInterpolationEnable"=w307:bool)
            n84 = case shown="True" w307 {
              tunnel: w313 -> [_ w321]
              tunnel: w312 -> [w315 w320]
              tunnel: [w315 w319] -> w311
              tunnel: w310 -> [_ w317]
              tunnel: [errorcluster {"status"=FALSE, "code"=0, "source"=""} ("error out") w316] -> w309
              frame False {
              }
              frame True {
                n85 = Unbundle By Name(w321) -> ("trajectoryInterpolationEnable"=w318:bool)
                n86 = call <vilib>:"CTRE_Phoenix_MotorControl_ConfigMotionProfileTrajectoryInterpolationEnable.vi"("timeoutMs"=w317, "enable?"=w318, "PhoenixMotorControlDevRef"=w320) -> ("error out"=w316:errorcluster, "PhoenixMotorControlDevRef"=w319:T7)  [unwired: 7 in]
              }
            }
          }
          frame 18 {
            n87 = Unbundle By Name(w323) -> ("feedbackNotContinuous"=w322:bool)
            n88 = case shown="True" w322 {
              tunnel: w328 -> [_ w336]
              tunnel: w327 -> [w330 w335]
              tunnel: [w330 w334] -> w326
              tunnel: w325 -> [_ w332]
              tunnel: [errorcluster {"status"=FALSE, "code"=0, "source"=""} ("error out") w331] -> w324
              frame False {
              }
              frame True {
                # "Configure Feedback Not Continuous"
                n89 = Unbundle By Name(w336) -> ("feedbackNotContinuous"=w333:bool)
                n90 = call <vilib>:"CTRE_Phoenix_MotorControl_ConfigFeedbackNotContinuous.vi"("timeoutMs"=w332, "FeedbackNotContinuous"=w333, "PhoenixMotorControlDevRef"=w335) -> ("error out"=w331:errorcluster, "PhoenixMotorControlDevRef"=w334:T7)  [unwired: 7 in]
              }
            }
          }
          frame 19 {
            # "Config Remote Sensor Closed Loop Disabled On Loss Of Signal"
            n91 = Unbundle By Name(w338) -> ("remoteSensorClosedLoopDisableNeutralOnLOS"=w337:bool)
            n92 = case shown="True" w337 {
              tunnel: w343 -> [_ w351]
              tunnel: w342 -> [w345 w350]
              tunnel: [w345 w349] -> w341
              tunnel: w340 -> [_ w347]
              tunnel: [errorcluster {"status"=FALSE, "code"=0, "source"=""} ("error out") w346] -> w339
              frame False {
              }
              frame True {
                n93 = Unbundle By Name(w351) -> ("remoteSensorClosedLoopDisableNeutralOnLOS"=w348:bool)
                n94 = call <vilib>:"CTRE_Phoenix_MotorControl_ConfigRemoteSensorClosedLoopDisableNeutralOnLOS.vi"("timeoutMs"=w347, "Disable Neutral on LOS"=w348, "PhoenixMotorControlDevRef"=w350) -> ("error out"=w346:errorcluster, "PhoenixMotorControlDevRef"=w349:T7)  [unwired: 7 in]
              }
            }
          }
          frame 20 {
            # "Configure Clear Position On Limit Forward"
            n95 = Unbundle By Name(w353) -> ("clearPositionOnLimitF"=w352:bool)
            n96 = case shown="True" w352 {
              tunnel: w358 -> [_ w366]
              tunnel: w357 -> [w360 w365]
              tunnel: [w360 w363] -> w356
              tunnel: w355 -> [_ w362]
              tunnel: [errorcluster {"status"=FALSE, "code"=0, "source"=""} ("error out") w361] -> w354
              frame False {
              }
              frame True {
                n97 = Unbundle By Name(w366) -> ("clearPositionOnLimitF"=w364:bool)
                n98 = call <vilib>:"CTRE_Phoenix_MotorControl_ConfigClearPositionOnLimitF.vi"("timeoutMs"=w362, "Clear Position On Limit F"=w364, "PhoenixMotorControlDevRef"=w365) -> ("error out"=w361:errorcluster, "PhoenixMotorControlDevRef"=w363:T7)  [unwired: 7 in]
              }
            }
          }
          frame 21 {
            # "Config Clear Position On Limit Reverse"
            n99 = Unbundle By Name(w368) -> ("clearPositionOnLimitR"=w367:bool)
            n100 = case shown="True" w367 {
              tunnel: w373 -> [_ w381]
              tunnel: w372 -> [w375 w379]
              tunnel: [w375 w378] -> w371
              tunnel: w370 -> [_ w377]
              tunnel: [errorcluster {"status"=FALSE, "code"=0, "source"=""} ("error out") w376] -> w369
              frame False {
              }
              frame True {
                n101 = Unbundle By Name(w381) -> ("clearPositionOnLimitR"=w380:bool)
                n102 = call <vilib>:"CTRE_Phoenix_MotorControl_ConfigClearPositionOnLimitR.vi"("timeoutMs"=w377, "Clear Position On Limit R"=w380, "PhoenixMotorControlDevRef"=w379) -> ("error out"=w376:errorcluster, "PhoenixMotorControlDevRef"=w378:T7)  [unwired: 7 in]
              }
            }
          }
          frame 22 {
            # "Configure Clear Position On Quad Index"
            n103 = Unbundle By Name(w383) -> ("clearPositionOnQuadIdx"=w382:bool)
            n104 = case shown="True" w382 {
              tunnel: w388 -> [_ w396]
              tunnel: w387 -> [w390 w395]
              tunnel: [w390 w394] -> w386
              tunnel: w385 -> [_ w392]
              tunnel: [errorcluster {"status"=FALSE, "code"=0, "source"=""} ("error out") w391] -> w384
              frame False {
              }
              frame True {
                n105 = Unbundle By Name(w396) -> ("clearPositionOnQuadIdx"=w393:bool)
                n106 = call <vilib>:"CTRE_Phoenix_MotorControl_ConfigClearPositionOnQuadIdx.vi"("timeoutMs"=w392, "Clear Position On Quad Idx"=w393, "PhoenixMotorControlDevRef"=w395) -> ("error out"=w391:errorcluster, "PhoenixMotorControlDevRef"=w394:T7)  [unwired: 7 in]
              }
            }
          }
          frame 23 {
            # "Config Limit Switch Disabled On Loss Of Signal"
            n107 = Unbundle By Name(w398) -> ("limitSwitchDisableNeutralOnLOS"=w397:bool)
            n108 = case shown="True" w397 {
              tunnel: w403 -> [_ w411]
              tunnel: w402 -> [w405 w409]
              tunnel: w401 -> [_ w408]
              tunnel: [w405 w407] -> w400
              tunnel: [errorcluster {"status"=FALSE, "code"=0, "source"=""} ("error out") w406] -> w399
              frame False {
              }
              frame True {
                n109 = Unbundle By Name(w411) -> ("limitSwitchDisableNeutralOnLOS"=w410:bool)
                n110 = call <vilib>:"CTRE_Phoenix_MotorControl_ConfigLimitSwitchDisableNeutralOnLOS.vi"("timeoutMs"=w408, "Disable Neutral On LOS"=w410, "PhoenixMotorControlDevRef"=w409) -> ("error out"=w406:errorcluster, "PhoenixMotorControlDevRef"=w407:T7)  [unwired: 7 in]
              }
            }
          }
          frame 24 {
            # "Config Soft Limit Disable Neutral On Loss Of Signal"
            n111 = Unbundle By Name(w413) -> ("softLimitDisableNeutralOnLOS"=w412:bool)
            n112 = case shown="True" w412 {
              tunnel: w418 -> [_ w426]
              tunnel: w417 -> [w420 w424]
              tunnel: [w420 w423] -> w416
              tunnel: w415 -> [_ w422]
              tunnel: [errorcluster {"status"=FALSE, "code"=0, "source"=""} ("error out") w421] -> w414
              frame False {
              }
              frame True {
                n113 = Unbundle By Name(w426) -> ("softLimitDisableNeutralOnLOS"=w425:bool)
                n114 = call <vilib>:"CTRE_Phoenix_MotorControl_ConfigSoftLimitDisableNeutralOnLOS.vi"("timeoutMs"=w422, "Soft Limit Disable Neutral On LOS"=w425, "PhoenixMotorControlDevRef"=w424) -> ("error out"=w421:errorcluster, "PhoenixMotorControlDevRef"=w423:T7)  [unwired: 7 in]
              }
            }
          }
          frame 25 {
            # "Config Pulse Width Edges Per Rotation"
            n115 = Unbundle By Name(w428) -> ("pulseWidthPeriod_EdgesPerRot"=w427:bool)
            n116 = case shown="True" w427 {
              tunnel: w433 -> [_ w441]
              tunnel: w432 -> [w435 w439]
              tunnel: [w435 w438] -> w431
              tunnel: [errorcluster {"status"=FALSE, "code"=0, "source"=""} ("error out") w437] -> w430
              tunnel: w429 -> [_ w436]
              frame False {
              }
              frame True {
                n117 = Unbundle By Name(w441) -> ("pulseWidthPeriod_EdgesPerRot"=w440:i32)
                n118 = call <vilib>:"CTRE_Phoenix_MotorControl_ConfigPulseWidthPeriod_EdgesPerRotation.vi"("timeoutMs"=w436, "Edges Per Rot"=w440, "PhoenixMotorControlDevRef"=w439) -> ("error out"=w437:errorcluster, "PhoenixMotorControlDevRef"=w438:T7)  [unwired: 7 in]
              }
            }
          }
          frame 26 {
            # "Config Pulse Width Filter Window Size"
            n119 = Unbundle By Name(w442) -> ("pulseWidthPeriod_FilterWindowSz"=w443:bool)
            n120 = case shown="True" w443 {
              tunnel: w448 -> [_ w456]
              tunnel: w447 -> [w450 w454]
              tunnel: [w450 w453] -> w446
              tunnel: w445 -> [_ w452]
              tunnel: [errorcluster {"status"=FALSE, "code"=0, "source"=""} ("error out") w451] -> w444
              frame False {
              }
              frame True {
                n121 = Unbundle By Name(w456) -> ("pulseWidthPeriod_FilterWindowSz"=w455:i32)
                n122 = call <vilib>:"CTRE_Phoenix_MotorControl_ConfigPulseWidthPeriod_FilterWindodwSz.vi"("timeoutMs"=w452, "Filter Window Size"=w455, "PhoenixMotorControlDevRef"=w454) -> ("error out"=w451:errorcluster, "PhoenixMotorControlDevRef"=w453:T7)  [unwired: 7 in]
              }
            }
          }
          frame 27 {
            n123 = Unbundle By Name(w464) -> ("customParam"=w460:T6)
            n124 = call <vilib>:"CTRE_Phoenix_MotorControl_ConfigAllCustomParameters.vi"("timeoutMs"=w461, "CustomParam"=w460, "PhoenixMotorControlDevRef in"=w463) -> ("AnyConfigFailed"=w458:bool, "PhoenixMotorControlDevRef out"=w462:T7)  [unwired: 7 in]
            n125 = Bundle By Name(cluster=errorcluster {"status"=FALSE, "code"=0, "source"=""} ("error out"), "status"=w458) -> (w457:errorcluster)
          }
          frame Default {
          }
        }
      }
      n126 = Or Array Elements(Boolean array=w20) -> (logical OR=w11:bool)
      n127 = Select(t=errorcluster {"status"=TRUE, "code"=-1, "source"="BaseMotorController Config All: One or more Configs failed"} ("error out 2"), s=w11, f=errorcluster {"status"=FALSE, "code"=0, "source"=""} ("error out 2")) -> (s? t:f=w8:errorcluster)
    }
    frame Error {
    }
  }
  "PhoenixMotorControlDevRef out" <- w6
  "error out" <- w1
